vi "Load Texture.vi"(11 "Texture Name":path) -> (3 "Texture":T1)   [LabVIEW 2020, in "Raster (FPGA).lvlib"]
uses:
  Raster (FPGA).lvlib
  Rectangle Dimensions.ctl
  Texture.ctl
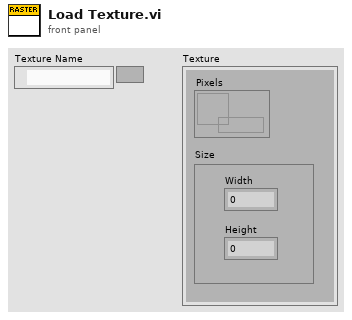
[diagram p1: front panel]
types:
  T1 = typedef "Raster (FPGA).lvlib/Texture.ctl" = cluster{"Pixels":refnum<data-value>, "Size":T2}
  T2 = typedef "Raster (FPGA).lvlib/Rectangle Dimensions.ctl" = cluster{"Width":u32, "Height":u32}
  T3 = typedef "imagedata.ctl" = cluster{"image type":i32, "image depth":i32, "image":u8[], "mask":u8[], "colors":u32[], "Rectangle":cluster{"left":i16, "top":i16, "right":i16, "bottom":i16}}
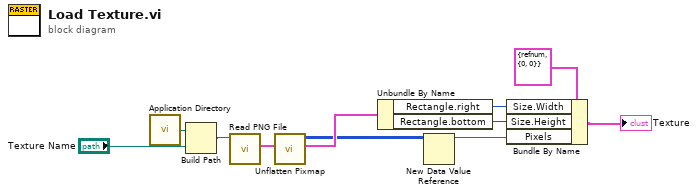
[diagram p0: block diagram]
diagram:
  n1 = call <vilib>:"Application Directory.vi"() -> ("Application Directory"=w3:path)
  n2 = Build Path(base path=w3, name or relative path="Texture Name") -> (appended path=w4:path)
  n3 = call <vilib>:"Read PNG File.vi"("path to PNG file"=w4) -> ("image data"=w6:T3)  [unwired: 8 in, 2 out]
  n4 = call <vilib>:"Unflatten Pixmap.vi"("image data"=w6) -> ("24-bit pixmap"=w1:u32[][])  [unwired: 4 in, 6 out]
  n5 = Unbundle By Name(w6) -> ("Rectangle.right"=w7:i16, "Rectangle.bottom"=w8:i16)
  n6 = New Data Value Reference(data value=w1) -> (data value reference=w5:refnum<data-value>)  [unwired: 1 in, 1 out]
  n7 = Bundle By Name(cluster=T1 {"Pixels"=refnum, "Size"={"Width"=0, "Height"=0}} ("Texture"), "Size.Width"=w7, "Size.Height"=w8, "Pixels"=w5) -> (→"Texture":T1)
